vi "系统矫正信息生成.vi"() -> ()   [LabVIEW 2018]
uses:
  <vilib>/vision/Calibration.llb/Error Statistics.ctl
  <vilib>/vision/Calibration.llb/Correction Learn Setup.ctl
  <vilib>/vision/Calibration.llb/Distortion Model Types.ctl
  <vilib>/vision/Calibration.llb/Distortion Model.ctl
  <vilib>/vision/NI_Vision_Development_Module.lvlib
panel:
  out "error out":errorcluster
  out "Calibration Axis Info":T1={"Origin Pixel"={"X"=0.0, "Y"=0.0}, "Angle Relative to Horizontal (deg)"=0.0, "X Axis Pixel"={"X"=0.0, "Y"=0.0}, "Axis Reference"=1} {"X Axis Pixel"."Y" format="%.2f"; "X Axis Pixel"."X" format="%.2f"; "Axis Reference" items=["Direct", "Indirect"]; "Angle Relative to Horizontal (deg)" format="%.2f"; "Origin Pixel"."Y" format="%.2f"; "Origin Pixel"."X" format="%.2f"}
  out "Grid Descriptor":T2={"X Step"=1.0, "Y Step"=1.0, "Unit"=enum."Undefined"} {"Y Step" format="%.2f"; "X Step" format="%.2f"}
  out "Calibration Learn Setup":T4={"Method"=4, "Distortion"=-1, "Corrected Image Scaling"=0, "Corrected Image Learn ROI"=0, "Learn Correction Table?"=FALSE} {"Distortion" items=["None"=-1, "Polynomial"=0, "Division"=1]; "Corrected Image Learn ROI" items=["Full Image ", "Calibration ROI", "ROI", "Calibration AND ROI", "Calibration OR ROI"]; "Corrected Image Scaling" items=["Scale to Preserve Area", "Scale to Fit"]; "Method" items=["Perspective", "Microplane", "Simple", "Corrected", "None"]}
  out "Error Statistics":T6
  out "Error Map":sgl[][](array[numeric]) format="%.2f"
  out "Image 2":T7(plugin-control)
  out "Image":T7(plugin-control)
  in  "路径":path
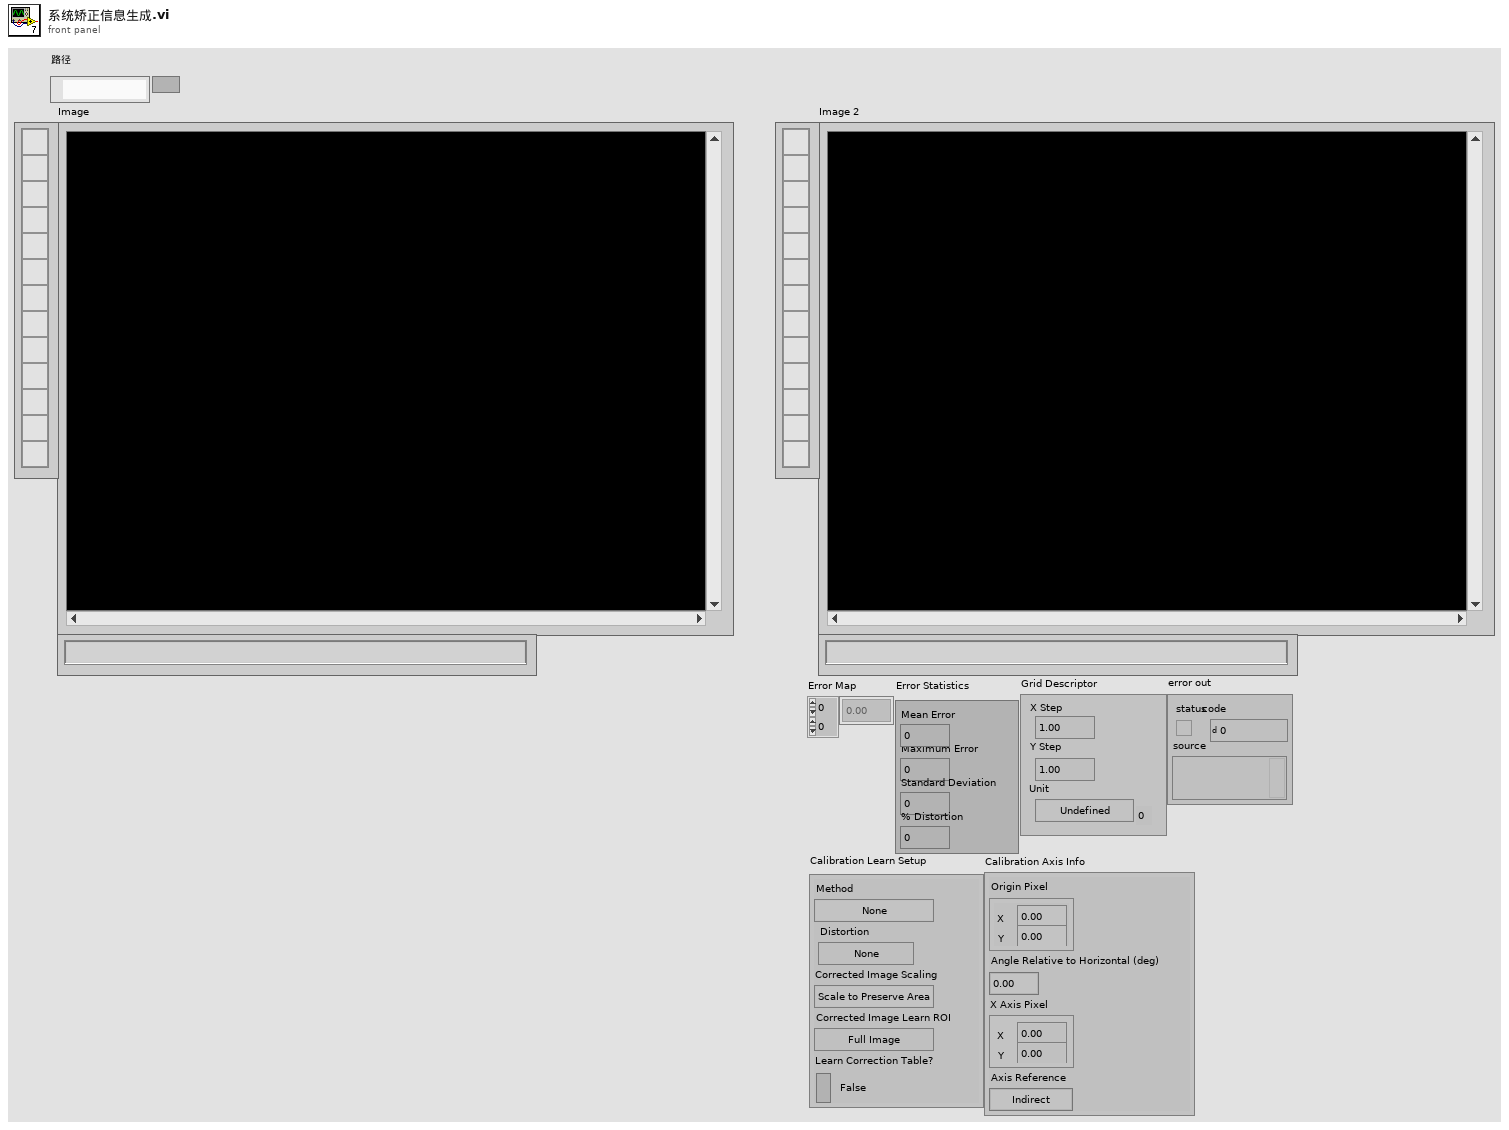
[diagram p1: front panel]
types:
  T1 = cluster{"Origin Pixel":cluster{"X":sgl, "Y":sgl}, "Angle Relative to Horizontal (deg)":sgl, "X Axis Pixel":cluster{"X":sgl, "Y":sgl}, "Axis Reference":u32}
  T2 = typedef "Simple Grid Descriptor" = cluster{"X Step":sgl, "Y Step":sgl, "Unit":T3}
  T3 = typedef "Image Unit" = enum32{"Undefined", "Angström", "Micrometer", "Millimeter", "Centimeter", "Meter", "Kilometer", "Microinch", "Inch", "Feet", "Nautical miles", "Standard miles", "Steps"}
  T4 = typedef "Correction Learn Setup.ctl" = cluster{"Method":u32, "Distortion":T5, "Corrected Image Scaling":u32, "Corrected Image Learn ROI":u32, "Learn Correction Table?":bool}
  T5 = typedef "Distortion Model Types.ctl" = i32
  T6 = typedef "Error Statistics.ctl" = cluster{"Mean Error":dbl, "Maximum Error":dbl, "Standard Deviation":dbl, "% Distortion":dbl}
  T7 = typedef "IMAQ Image.ctl" = refnum<image>
  T8 = typedef "Image Type" = u32
  T9 = typedef "Distortion Model.ctl" = cluster{"Distortion Model":T5, "Polynomial Model Setup":cluster{"Radial Coefficient":u32, "Tangential Coefficients ":bool}}
  T10 = typedef "Calibration Reference Points.ctl" = cluster{"Pixel Coordinates":cluster{"X":dbl, "Y":dbl}[], "Real World Coordinates":cluster{"X":dbl, "Y":dbl}[], "Unit":T3, "Image Size":cluster{"X":u32, "Y":u32}}
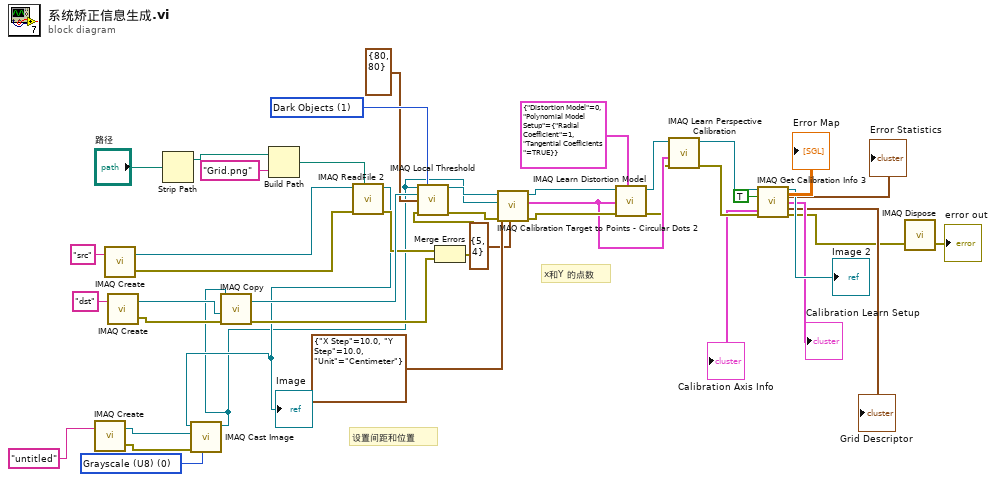
[diagram p0: block diagram]
diagram:
  w3 = T8 0 items=["Grayscale (U8)", "Grayscale (I16)", "Grayscale (SGL)", "Complex (CSG)", "RGB (U32)", "HSL (U32)", "RGB (U64)", "Grayscale (U16)"] ("Image Type")
  w32 = u32 1 items=["Bright Objects", "Dark Objects"] ("Look For (Bright Objects)")
  # "x和Y 的点数"
  # "设置间距和位置"
  n1 = call "IMAQ Create"("Image Name"="untitled") -> ("New Image"=w5:T7, "error out"=w6:errorcluster)  [unwired: 4 in]
  n2 = call "IMAQ Create"("Image Name"="src") -> ("New Image"=w39:T7, "error out"=w37:errorcluster)  [unwired: 4 in]
  n3 = call "IMAQ Create"("Image Name"="dst") -> ("New Image"=w34:T7, "error out"=w35:errorcluster)  [unwired: 4 in]
  n4 = Strip Path(path="路径") -> (stripped path=w42:path)  [unwired: 1 out]
  n5 = Build Path(base path=w42, name or relative path="Grid.png" ("名称或相对路径")) -> (appended path=w40:path)
  n6 = call "IMAQ ReadFile 2"("File Path"=w40, "error in (no error)"=w37, "Image"=w39) -> ("error out"=w31:errorcluster, "Image Out"=w4:T7)  [unwired: 4 in, 3 out]
  "Image" <- w4
  n7 = call "IMAQ Cast Image"("Image Type"=w3, "error in (no error)"=w6, "Image Dst"=w5, "Image Src"=w4) -> ("Image Dst Out"=w2:T7)  [unwired: 6 in, 1 out]
  n8 = call "IMAQ Copy"("error in (no error)"=w35, "Image Dst"=w34, "Image Src"=w2) -> ("error out"=w30:errorcluster, "Image Dst Out"=w33:T7)  [unwired: 3 in]
  n9 = Merge Errors(w31, w30) -> (w29:errorcluster)
  n10 = call "IMAQ Local Threshold"("Image Src"=w2, "Look For (Bright Objects)"=w32, "Image Dst"=w33, "Window Size (32x32)"=cluster{"SizeX":i32, "SizeY":i32} {"SizeX"=80, "SizeY"=80}, "error in (no error)"=w29) -> ("Image Dst Out"=w27:T7, "error out"=w25:errorcluster)  [unwired: 9 in]
  n11 = call "IMAQ Calibration Target to Points - Circular Dots 2"("Grid Size"=cluster{"Max X":u32, "Max Y":u32} {"Max X"=5, "Max Y"=4}, "error in (no error)"=w25, "Grid Descriptor"=cluster{"X Step":sgl, "Y Step":sgl, "Unit":T3} {"X Step"=10.0, "Y Step"=10.0, "Unit"=enum."Centimeter"}, "Grayscale Image"=w2, "Target Image"=w27) -> ("error out"=w22:errorcluster, "Reference Points"=w19:T10, "Target Image (dup)"=w23:T7)  [unwired: 4 in]
  n12 = call "IMAQ Learn Distortion Model"("Distortion Model Setup"=T9 {"Distortion Model"=0, "Polynomial Model Setup"={"Radial Coefficient"=1, "Tangential Coefficients "=TRUE}}, "error in (no error)"=w22, "Reference Points"=w19, "Calibration Template Image"=w23) -> ("error out"=w18:errorcluster, "Calibration Template Image Out"=w20:T7)  [unwired: 6 in]
  n13 = call "IMAQ Learn Perspective Calibration"("error in (no error)"=w18, "Reference Points"=w19, "Calibration Template Image"=w20) -> ("error out"=w16:errorcluster, "Calibration Template Image Out"=w17:T7)  [unwired: 7 in]
  n14 = call "IMAQ Get Calibration Info 3"("Calibration Template Image"=w17, "Return Error Information (False)"=TRUE, "error in (no error)"=w16) -> ("Error Map"=→"Error Map":sgl[][], "Calibration Template Image (duplicate)"=→"Image 2":T7, "Error Statistics"=→"Error Statistics":T6, "Calibration Learn Setup"=→"Calibration Learn Setup":T4, "Grid Descriptor"=→"Grid Descriptor":T2, "Calibration Axis Info"=→"Calibration Axis Info":T1, "error out"=w10:errorcluster)  [unwired: 4 in, 2 out]
  n15 = call "IMAQ Dispose"("error in (no error)"=w10) -> ("error out"=→"error out":errorcluster)  [unwired: 5 in]
